vi "Acquisition Settings Dialog.vi"(8 "error in (no error)":errorcluster, 11 "Tasks in":T1[](array[typedef])) -> (0 "error out":errorcluster, 2 "cancelled":bool, 3 "Tasks out":T1[](array[typedef]))   [LabVIEW 2018, in "DAQ Write.lvlib"]
uses:
  Task Cluster (with Add Remove Buttons).ctl
  Task Cluster.ctl
  DAQ/DAQ Write Folder/DAQ/DAQ Write.lvlib
  DAQ/DAQ.lvlib
panel:
  in  "Cancel Button":bool
  in  "OK Button":bool
  in  "Task List":T2[](array[typedef]) caption="Channel List"
  # "DAQmx Tasks"
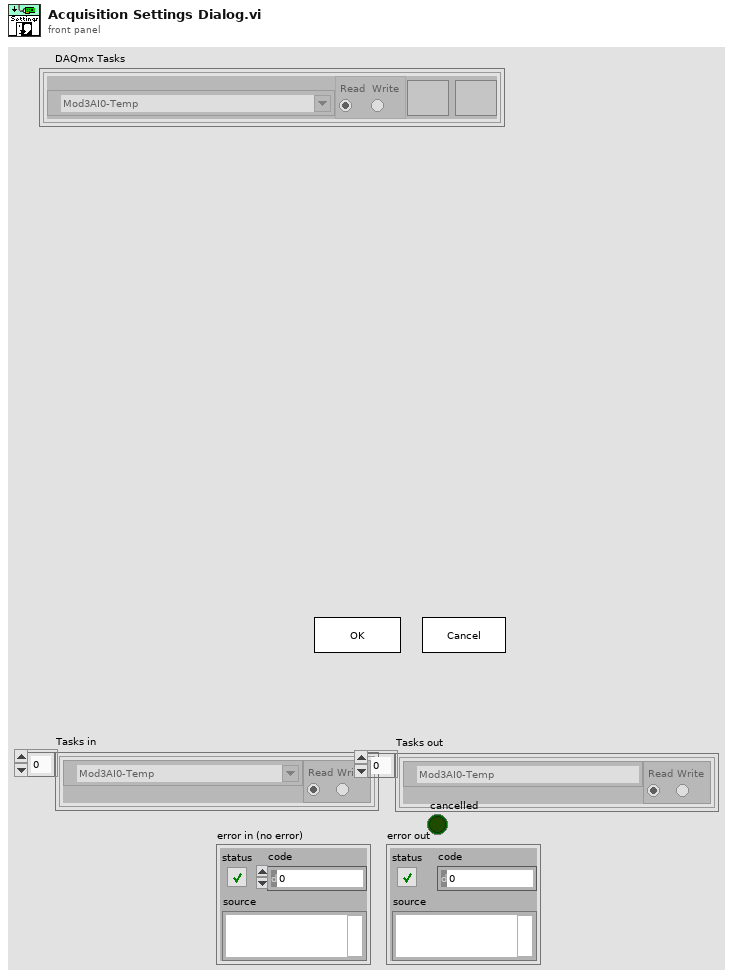
[diagram p1: front panel]
types:
  T1 = typedef "Task Cluster.ctl" = cluster{"DAQmx Task":refnum<k21>, "Read-Write Radio":enum32{"Read", "Write"}}
  T2 = typedef "DAQ.lvlib/Task Cluster (with Add Remove Buttons).ctl" = cluster{"Add Button":bool, "Remove Button":bool, "DAQmx Task":refnum<k21>, "Radio Buttons":enum32{"Read", "Write"}}
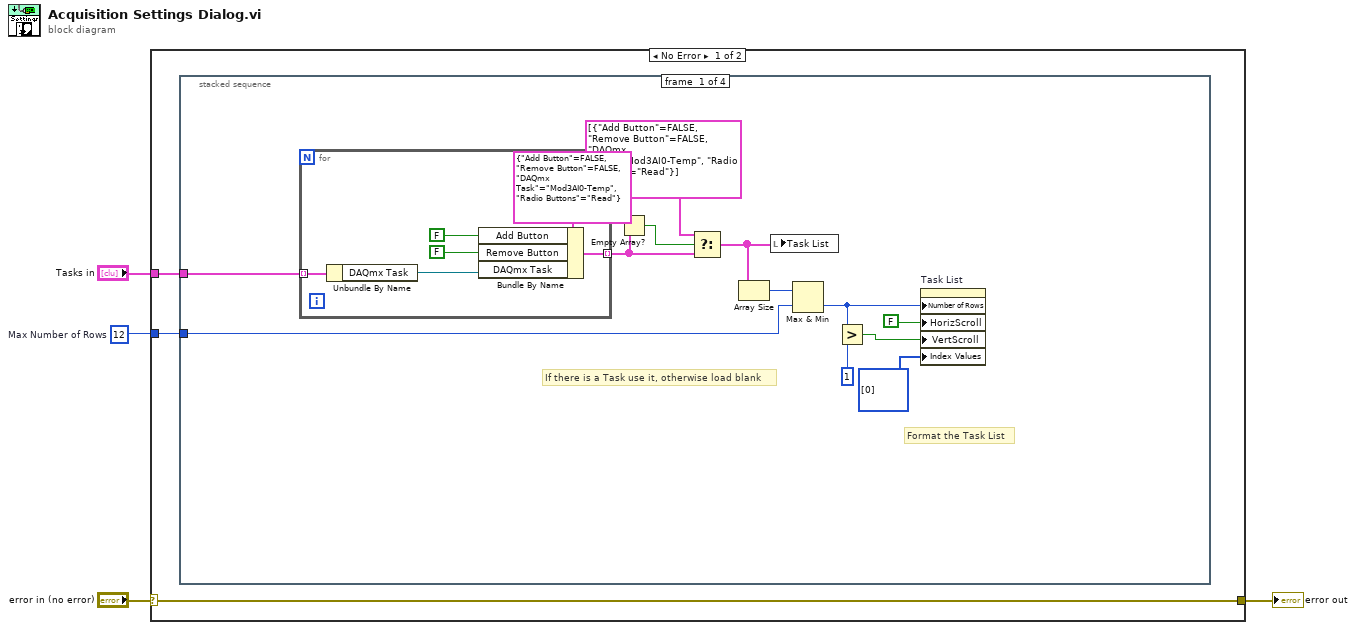
[diagram p0: block diagram]
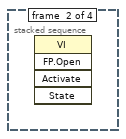
[diagram p2: hidden frame]
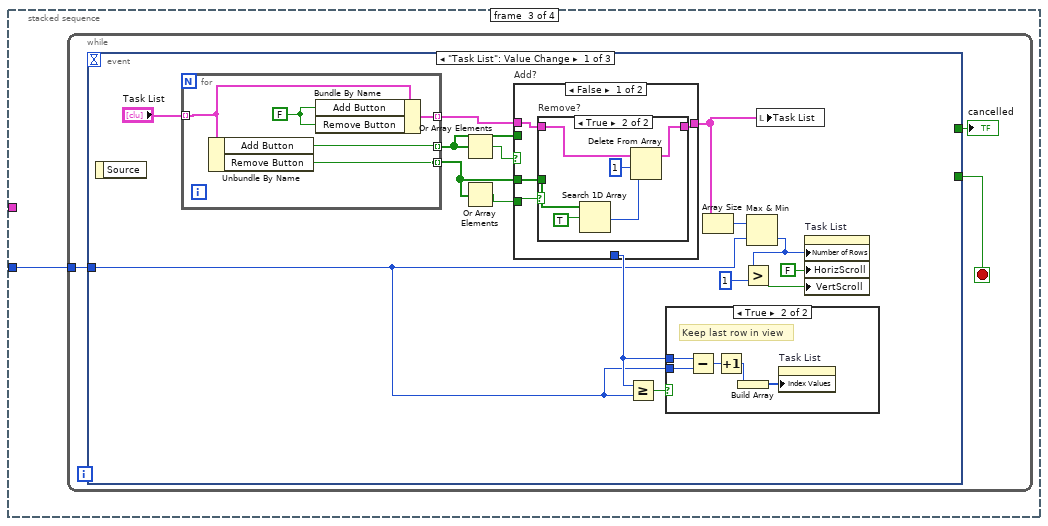
[diagram p3: hidden frame]
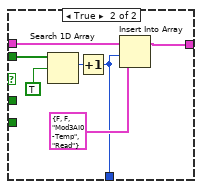
[diagram p6: hidden frame]
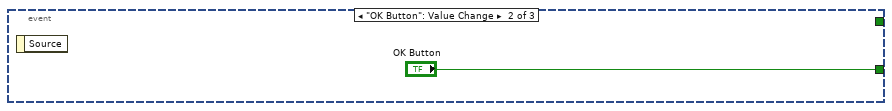
[diagram p7: hidden frame]
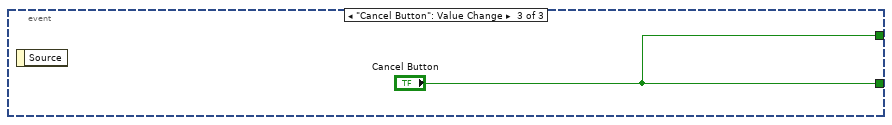
[diagram p8: hidden frame]
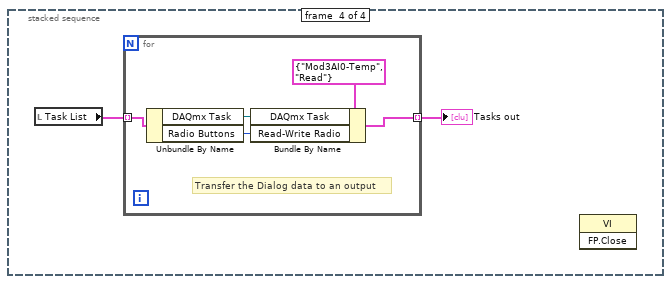
[diagram p9: hidden frame]
diagram:
  w1 = u32 12  # Max Number of Rows
  n1 = case shown="No Error" "error in (no error)" {
    selector: "error in (no error)" -> [w7 w82]
    tunnel: [w7 w82] -> w3
    tunnel: "Tasks in" -> [w6 _]
    tunnel: w1 -> [w5 _]
    frame No Error {
      n2 = stacked-sequence {
        tunnel: w6 -> [w19 _ _ _]
        tunnel: w5 -> [w13 _ w26 _]
        frame #0 {
          # "Format the Task List"
          # "If there is a Task use it, otherwise load blank"
          n3 = for {
            tunnel: w19 -> [w25] mode=indexing
            tunnel: [w20] -> w16 mode=indexing
            n4 = Unbundle By Name(w25) -> ("DAQmx Task"=w22:refnum<k21>)
            n5 = Bundle By Name(cluster=T2 {"Add Button"=FALSE, "Remove Button"=FALSE, "DAQmx Task"="Mod3AI0-Temp", "Radio Buttons"=enum."Read"} ("DAQmx Channel Cluster"), "Add Button"=FALSE, "Remove Button"=FALSE, "DAQmx Task"=w22) -> (w20:T2)
          }
          n6 = Empty Array?(array=w16) -> (empty?=w18:bool)
          n7 = Select(t=T2[] [{"Add Button"=FALSE, "Remove Button"=FALSE, "DAQmx Task"="Mod3AI0-Temp", "Radio Buttons"=enum."Read"}] ("Channel List"), s=w18, f=w16) -> (s? t:f=w15:T2[])
          n8 = Array Size(array=w15) -> (size(s)=w14:i32)
          n9 = local write "Task List"(w15) -> ()
          n10 = Max & Min(x=w14, y=w13) -> (min(x,y)=w11:u32)  [unwired: 1 out]
          n11 = Greater?(x=w11, y=u32 1) -> (0:w9:bool)
          n12 = property on="Task List" class="Arr"("Number of Rows"=w11, "HorizScroll"=FALSE ("Horizontal Scrollbar Visible"), "VertScroll"=w9, "Index Values"=u32[] [0]) -> ()  [unwired: 2 in, 2 out]
        }
        frame #1 {
          n13 = invoke class="VI" method="FP.Open"() -> ()  [unwired: 5 in, 5 out]
        }
        frame #2 {
          n14 = while {
            tunnel: w26 -> [w29]
            stop <- w28 stop-if-true
            n15 = event shown="[0] \"Task List\": Value Change" {
              selector: _ -> [_ _ _]
              dyn-events: _ -> [_ _ _]
              timeout: _ -> [_ _ _]
              tunnel: [_ "OK Button" "Cancel Button"] -> w28
              tunnel: w29 -> [w30 _ _]
              tunnel: [_ _ "Cancel Button"] -> w27
              event "Task List": Value Change {
                n16 = event-data() -> ()  [unwired: 1 in, 1 out]
                n17 = for {
                  tunnel: "Task List" -> [w71] mode=indexing
                  tunnel: [w68] -> w42 mode=indexing
                  tunnel: [w72] -> w40 mode=indexing
                  tunnel: [w69] -> w41 mode=indexing
                  w70 = FALSE ("Add Button")
                  n18 = Unbundle By Name(w71) -> ("Add Button"=w68:bool, "Remove Button"=w72:bool)
                  n19 = Bundle By Name(cluster=w71, "Add Button"=w70, "Remove Button"=w70) -> (w69:T2)
                }
                n20 = Or Array Elements(Boolean array=w42) -> (logical OR=w43:bool)
                n21 = Or Array Elements(Boolean array=w40) -> (logical OR=w39:bool)
                n22 = case "Add?" shown="False" w43 {
                  tunnel: w42 -> [_ w67]
                  tunnel: w41 -> [w51 w65]
                  tunnel: [w50 w62] -> w38
                  tunnel: w40 -> [w53 _]
                  tunnel: w39 -> [w52 _]
                  tunnel: [_ w61] -> w31
                  frame False {
                    n23 = case "Remove?" shown="True" w52 {
                      tunnel: w53 -> [_ w59]
                      tunnel: w51 -> [w54 w58]
                      tunnel: [w54 w55] -> w50
                      frame False {
                      }
                      frame True {
                        n24 = Search 1D Array(1D array=w59, element=TRUE) -> (index of element=w56:i32)  [unwired: 1 in]
                        n25 = Delete From Array(array=w58, length=1, index=w56) -> (array with subset deleted=w55:T2[])  [unwired: 1 out]
                      }
                    }
                  }
                  frame True {
                    n26 = Search 1D Array(1D array=w67, element=TRUE) -> (index of element=w64:i32)  [unwired: 1 in]
                    n27 = Increment(x=w64) -> (x+1=w61:i32)
                    n28 = Insert Into Array(array=w65, index=w61, new element=T2 {"Add Button"=FALSE, "Remove Button"=FALSE, "DAQmx Task"="Mod3AI0-Temp", "Radio Buttons"=enum."Read"} ("new element/subarray")) -> (w62:T2[])
                  }
                }
                n29 = Greater Or Equal?(x=w31, y=w30) -> (x >= y?=w32:bool)
                n30 = case shown="True" w32 {
                  tunnel: w31 -> [_ w49]
                  tunnel: w30 -> [_ w48]
                  frame False {
                  }
                  frame True {
                    # "Keep last row in view"
                    n31 = Subtract(x=w49, y=w48) -> (x-y=w47:u32)
                    n32 = Increment(x=w47) -> (x+1=w45:u32)
                    n33 = Build Array(w45) -> (w46:u32[])
                    n34 = property on="Task List" class="Arr"("Index Values"=w46) -> ()  [unwired: 2 in, 2 out]
                  }
                }
                n35 = Array Size(array=w38) -> (size(s)=w37:i32)
                n36 = Max & Min(x=w37, y=w30) -> (min(x,y)=w34:u32)  [unwired: 1 out]
                n37 = Greater?(x=w34, y=u32 1) -> (0:w33:bool)
                n38 = local write "Task List"(w38) -> ()
                n39 = property on="Task List" class="Arr"("Number of Rows"=w34, "HorizScroll"=FALSE ("Horizontal Scrollbar Visible"), "VertScroll"=w33) -> ()  [unwired: 2 in, 2 out]
              }
              event "OK Button": Value Change {
                n40 = event-data() -> ()  [unwired: 1 in, 1 out]
              }
              event "Cancel Button": Value Change {
                n41 = event-data() -> ()  [unwired: 1 in, 1 out]
              }
            }
            "cancelled" <- w27
          }
        }
        frame #3 {
          n42 = local read "Task List"() -> (w76:T2[])
          n43 = for {
            tunnel: w76 -> [w81] mode=indexing
            tunnel: [w79] -> w75 mode=indexing
            # "Transfer the Dialog data to an output"
            n44 = Unbundle By Name(w81) -> ("DAQmx Task"=w80:refnum<k21>, "Radio Buttons"=w77:enum32{"Read", "Write"})
            n45 = Bundle By Name(cluster=T1 {"DAQmx Task"="Mod3AI0-Temp", "Read-Write Radio"=enum."Read"} ("DAQmx Channel Cluster"), "DAQmx Task"=w80, "Read-Write Radio"=w77) -> (w79:T1)
          }
          "Tasks out" <- w75
          n46 = invoke class="VI" method="FP.Close"() -> ()  [unwired: 3 in, 3 out]
        }
      }
    }
    frame Error {
    }
  }
  "error out" <- w3
